vi "Get State.vi"(8 "error in (no error)":errorcluster, 11 "Timer in":refnum<class "Timer.lvclass">) -> (0 "error out":errorcluster, 1 "Result ready":bool, 2 "Armed":bool, 3 "Timer out":refnum<class "Timer.lvclass">, 4 "Check again":bool)   [LabVIEW 2018, in "Timer.lvclass"]
uses:
  Timer.lvclass
  C:/github/2018/LabActor/Worker/Worker.lvclass
  Timer.lvclass/Timer.ctl
  Worker/Worker.lvclass/Worker.ctl
  Write Delay active.vi
  Worker/Write Check again delay.vi
  Read Delay active.vi
  Worker/Worker.lvclass
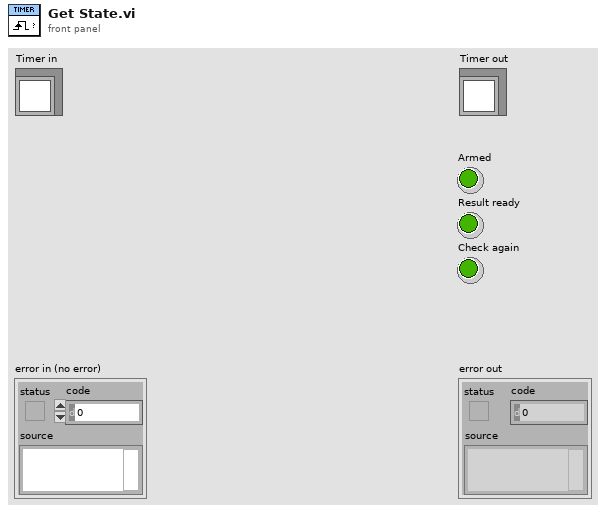
[diagram p1: front panel]
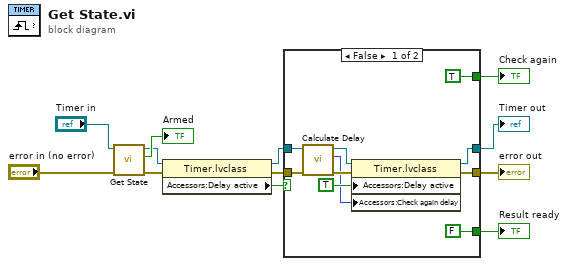
[diagram p0: block diagram]
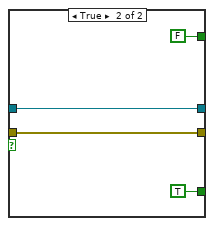
[diagram p2: hidden frame]
diagram:
  n1 = call-parent "Get State.vi"("error in (no error)"="error in (no error)", "Worker in"="Timer in") -> ("error out"=w12:errorcluster, "Armed"=→"Armed":bool, "Worker out"=w8:refnum<class "Timer.lvclass">)  [unwired: 5 in, 2 out]
  n2 = property class="Timer.lvclass"(reference=w8, error in=w12) -> (reference out=w6:refnum<class "Timer.lvclass">, error out=w5:errorcluster, "Accessors:Delay active"=w7:bool)
  n3 = case shown="False" w7 {
    tunnel: w6 -> [w22 w26]
    tunnel: w5 -> [w18 w25]
    tunnel: [w16 w26] -> w4
    tunnel: [TRUE ("Delay active") FALSE ("Delay active")] -> w3
    tunnel: [FALSE ("Delay active") TRUE ("Delay active")] -> w2
    tunnel: [w13 w25] -> w1
    frame False {
      n4 = call-dynamic "Calculate Delay.vi"("error in (no error)"=w18, "Timer in"=w22) -> ("error out"=w20:errorcluster, "Delay"=w17:i32, "Timer out"=w21:refnum<class "Timer.lvclass">)  [unwired: 7 in]
      n5 = property class="Timer.lvclass"(reference=w21, error in=w20, "Accessors:Delay active"=TRUE ("Delay active"), "Accessors:Check again delay"=w17) -> (reference out=w16:refnum<class "Timer.lvclass">, error out=w13:errorcluster)
    }
    frame True {
    }
  }
  "error out" <- w1
  "Timer out" <- w4
  "Result ready" <- w2
  "Check again" <- w3
